vi "Pure Pursuit Velocity FF.vi"(5 "kffa":dbl, 7 "kffv":dbl, 8 "dt":dbl format="%0.2f", 9 "Odometry":T1, 10 "Right Desired Velocity":dbl, 11 "Left Desired Velocity":dbl) -> (2 "Right Velocity":dbl, 3 "Left Velocity":dbl)   [LabVIEW 2017, in "Pure Pursuit.lvlib"]
uses:
  Pure Pursuit.lvlib
  Odometry/Typedef/Odometry.ctl
  <vilib>/ptbypt/NI_PtbyPt.lvlib
panel:
  in  "reinitialize?":bool
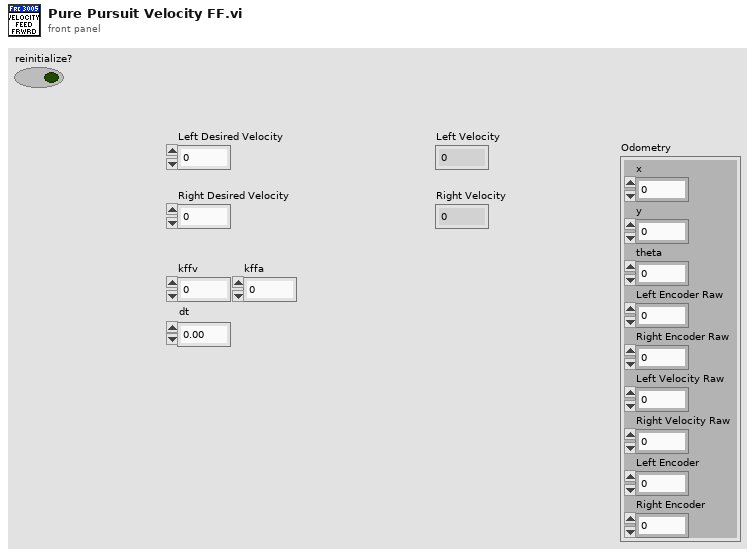
[diagram p1: front panel]
types:
  T1 = typedef "Odometry.ctl" = cluster{"x":dbl, "y":dbl, "theta":dbl, "Left Encoder Raw":i32, "Right Encoder Raw":i32, "Left Velocity Raw":i32, "Right Velocity Raw":i32, "Left Encoder":dbl, "Right Encoder":dbl}
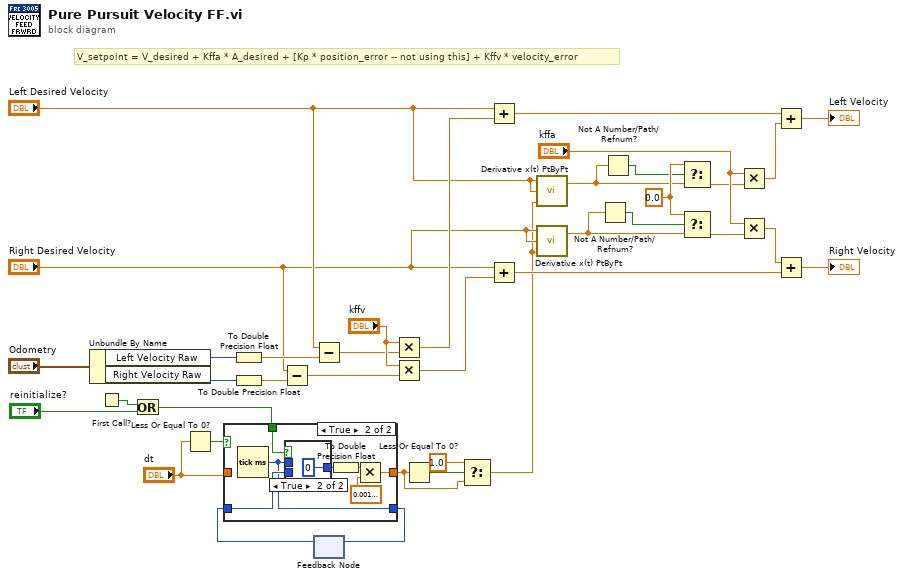
[diagram p0: block diagram]
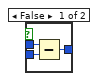
[diagram p3: hidden frame]
diagram:
  w9 = 0.0 ("t")
  # "V_setpoint = V_desired + Kffa * A_desired + [Kp * position_error -- not using this] + Kffv * velocity_error"
  n1 = Unbundle By Name("Odometry") -> ("Left Velocity Raw"=w36:i32, "Right Velocity Raw"=w34:i32)
  n2 = First Call?() -> (First Call?: T/F=w16:bool)
  n3 = Or(x=w16, y="reinitialize?") -> (x .or. y?=w17:bool)
  n4 = Less Or Equal To 0?(x="dt") -> (x <= 0?=w14:bool)
  n5 = To Double Precision Float(number=w36) -> (double precision float=w35:dbl)
  n6 = To Double Precision Float(number=w34) -> (double precision float=w33:dbl)
  n7 = Subtract(x="Right Desired Velocity", y=w33) -> (x-y=w21:dbl)
  n8 = Subtract(x="Left Desired Velocity", y=w35) -> (x-y=w22:dbl)
  n9 = feedback #1() -> (w19:u32)  [unwired: 1 in]
  n10 = case shown="True" w14 {
    tunnel: [w39 w43] -> w1
    tunnel: w19 -> [w38 w42]
    tunnel: [w38 w41] -> w20
    tunnel: "dt" -> [w39 _]
    tunnel: w17 -> [_ w40]
    frame False {
    }
    frame True {
      n11 = Tick Count (ms)() -> (millisecond timer value=w41:u32)
      n12 = case shown="True" w40 {
        tunnel: [w49 u32 0] -> w45
        tunnel: w42 -> [w48 _]
        tunnel: w41 -> [w47 _]
        frame False {
          n13 = Subtract(x=w47, y=w48) -> (x-y=w49:u32)
        }
        frame True {
        }
      }
      n14 = To Double Precision Float(number=w45) -> (double precision float=w44:dbl)
      n15 = Multiply(x=w44, y=0.0010000000474974513) -> (x*y=w43:dbl)
    }
  }
  n16 = feedback-in #1(w20) -> ()
  n17 = Multiply(x="kffv", y=w22) -> (x*y=w29:dbl)
  n18 = Multiply(x="kffv", y=w21) -> (x*y=w28:dbl)
  n19 = Less Or Equal To 0?(x=w1) -> (x <= 0?=w3:bool)
  n20 = Select(t=1.0, s=w3, f=w1) -> (s? t:f=w4:dbl)
  n21 = Add(x="Left Desired Velocity", y=w29) -> (x+y=w32:dbl)
  n22 = Add(x="Right Desired Velocity", y=w28) -> (x+y=w30:dbl)
  n23 = call <vilib>:"Derivative x(t) PtByPt.vi"("dt"=w4, "initial condition"="Left Desired Velocity", "x"="Left Desired Velocity") -> ("dx/dt"=w8:dbl)  [unwired: 1 in, 1 out]
  n24 = call <vilib>:"Derivative x(t) PtByPt.vi"("dt"=w4, "initial condition"="Right Desired Velocity", "x"="Right Desired Velocity") -> ("dx/dt"=w11:dbl)  [unwired: 1 in, 1 out]
  n25 = Not A Number/Path/Refnum?(number/path/refnum=w11) -> (NaN/Path/Refnum?=w10:bool)
  n26 = Not A Number/Path/Refnum?(number/path/refnum=w8) -> (NaN/Path/Refnum?=w7:bool)
  n27 = Select(t=w9, s=w7, f=w8) -> (s? t:f=w13:dbl)
  n28 = Select(t=w9, s=w10, f=w11) -> (s? t:f=w12:dbl)
  n29 = Multiply(x="kffa", y=w13) -> (x*y=w25:dbl)
  n30 = Multiply(x="kffa", y=w12) -> (x*y=w23:dbl)
  n31 = Add(x=w32, y=w25) -> (x+y=→"Left Velocity":dbl)
  n32 = Add(x=w23, y=w30) -> (x+y=→"Right Velocity":dbl)
